vi "Initialize (Control).vi"(5 "Password":string, 6 "Connect Timeout (4000 ms)":u32=4000, 7 "User Name":string, 8 "error in (no error)":errorcluster, 9 "Language (Automatic)":T1 items=["Automatic"=0, "Chinese Simplified"=2052, "English"=1033, "French"=1036, "German"=1031, "Japanese"=1041, "Korean"=1042], 10 "Force Property Refresh (T)":bool=TRUE, 11 "Target (localhost)":refnum<k21>="localhost") -> (0 "error out":errorcluster, 2 "Supported Experts":T2[](array[typedef]), 3 "Session out":refnum<k21>)   [LabVIEW 2017, in "nisyscfg.lvlib"]
uses:
  <vilib>/nisyscfg/nisyscfg.lvlib
  <vilib>/nisyscfg/Expert Info.ctl
  <vilib>/nisyscfg/Language.ctl
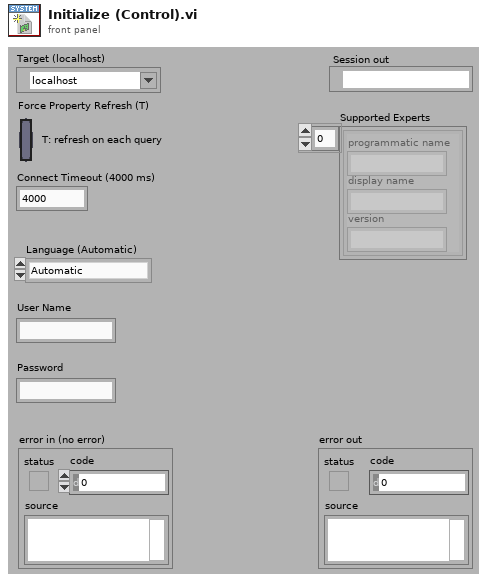
[diagram p1: front panel]
types:
  T1 = typedef "nisyscfg.lvlib/Language.ctl" = i32
  T2 = typedef "nisyscfg.lvlib/Expert Info.ctl" = cluster{"programmatic name":string, "display name":string, "version":string}
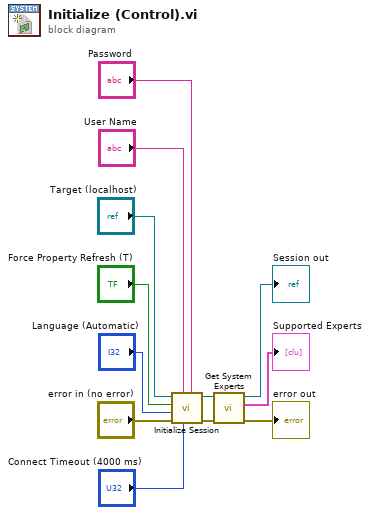
[diagram p0: block diagram]
diagram:
  n1 = call <vilib>:"Initialize Session.vi"("Password"="Password", "Connect Timeout (4000 ms)"="Connect Timeout (4000 ms)", "User Name"="User Name", "error in (no error)"="error in (no error)", "Language (Automatic)"="Language (Automatic)", "Force Property Refresh (T)"="Force Property Refresh (T)", "Target (localhost)"="Target (localhost)") -> ("error out"=w11:errorcluster, "Session out"=w8:refnum<k21>)  [unwired: 3 in]
  n2 = call <vilib>:"Get System Experts.vi"("error in (no error)"=w11, "Session in"=w8) -> ("error out"=→"error out":errorcluster, "Supported Experts"=→"Supported Experts":T2[], "Session out"=→"Session out":refnum<k21>)  [unwired: 7 in]
